vi "runtest Split AutoInc String.vi"(11 "Auto Inc Field Value":string) -> (0 "Use zero width?":bool, 1 "Width":i32, 2 "Increment Value":string, 3 "Auto Inc Field Prefix":string, 4 "# Preceding zeros":i32, 5 "Prefix without zero pad":string)   [LabVIEW 2011]
panel:
  out "Zeros match":string
  out "match substring":string
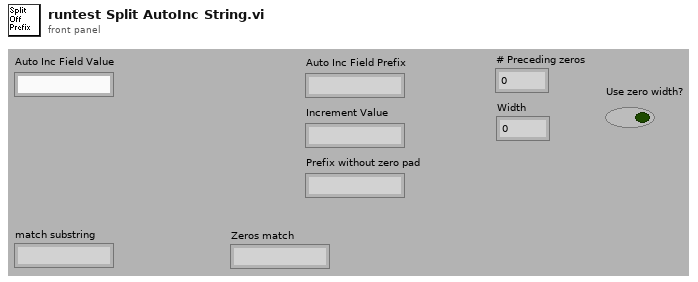
[diagram p1: front panel]
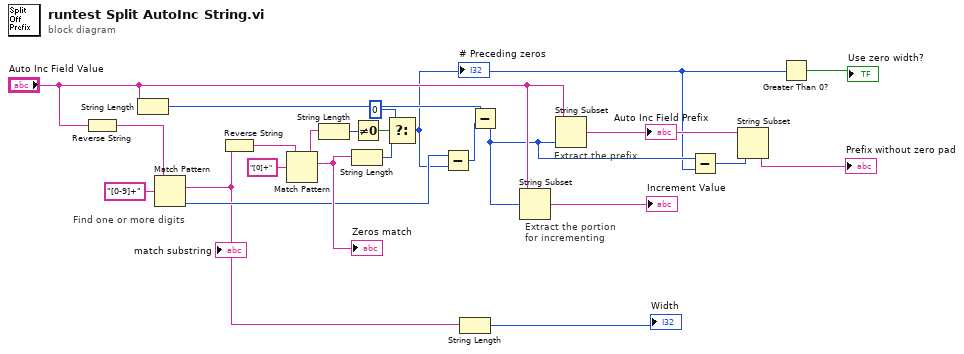
[diagram p0: block diagram]
diagram:
  # "Extract the prefix"
  # "Extract the portion\nfor incrementing"
  # "Find one or more digits"
  n1 = Reverse String(1:"Auto Inc Field Value") -> (0:w23:string)
  n2 = String Length(string="Auto Inc Field Value") -> (length=w21:i32)
  n3 = Match Pattern(string=w23, regular expression="[0-9]+") -> (match substring=w13:string, offset past match=w15:i32)  [unwired: 3 out]
  "match substring" <- w13
  n4 = Reverse String(1:w13) -> (0:w17:string)
  n5 = Match Pattern(string=w17, regular expression="[0]+") -> (before substring=w10:string, match substring=w16:string)  [unwired: 3 out]
  "Zeros match" <- w16
  n6 = String Length(string=w10) -> (length=w9:i32)
  n7 = String Length(string=w16) -> (length=w7:i32)
  n8 = Not Equal To 0?(x=w9) -> (x != 0?=w8:bool)
  n9 = Select(t=0, s=w8, f=w7) -> (s? t:f=w3:i32)
  "# Preceding zeros" <- w3
  n10 = Subtract(x=w15, y=w3) -> (x-y=w14:i32)
  n11 = String Length(string=w13) -> (length=→"Width":i32)
  n12 = Subtract(x=w21, y=w14) -> (x-y=w4:i32)
  n13 = String Subset(string="Auto Inc Field Value", offset (0)=w4) -> (substring=→"Increment Value":string)  [unwired: 1 out]
  n14 = String Subset(string="Auto Inc Field Value", length (rest)=w4) -> (substring=w5:string)  [unwired: 1 out]
  "Auto Inc Field Prefix" <- w5
  n15 = Subtract(x=w4, y=w3) -> (x-y=w2:i32)
  n16 = String Subset(string=w5, length (rest)=w2) -> (substring=→"Prefix without zero pad":string)  [unwired: 1 out]
  n17 = Greater Than 0?(x=w3) -> (x > 0?=→"Use zero width?":bool)
